vi "Keysight_ATI40_5.vi"() -> ()   [LabVIEW 2023]
uses:
  <vilib>/Analysis/baseanly.llb/A x Vector.vi
  <vilib>/Utility/file.llb/Write To Spreadsheet File (DBL).vi
  <instrlib>/Agilent 34970/Agilent 34970.lvlib
  <vilib>/Analysis/NI_AALBase.lvlib
panel:
  in  "Transform":T1
  in  "Torque Units":string="N-m"
  in  "Force Units":string="N"
  in  "Calibration File":path=path "C:/Users/d066566/OneDrive - Politecnico di Torino/PhD/PhD/Test files/Denver/FT17838/FT17838.cal"
  out "Output Number Array":dbl[](array[numeric]) format="%.2f"
  out "error out":errorcluster
  in  "Save":bool
  in  "Data File":path=path "C:/Users/d066566/Desktop/asdf3.csv"
  in  "Data format and type":string="%.6f"
  in  "stop":bool
  in  "VISA resource name":refnum<visa-resource-name>="GPIB0::9::INSTR"
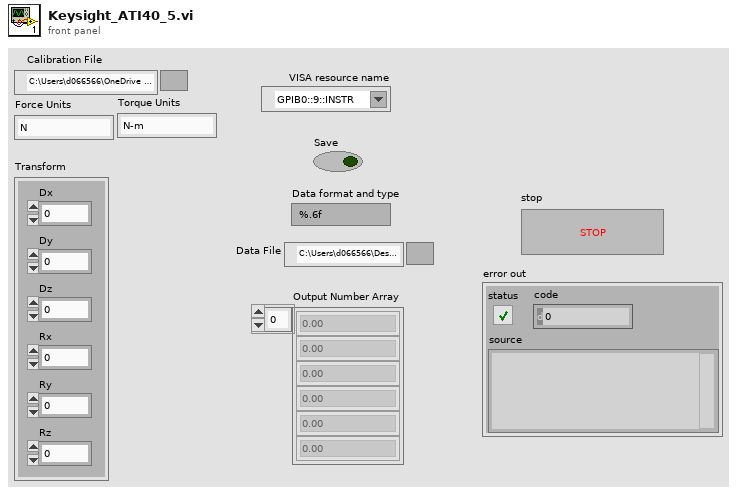
[diagram p1: front panel]
types:
  T1 = cluster{"Dx":dbl, "Dy":dbl, "Dz":dbl, "Rx":dbl, "Ry":dbl, "Rz":dbl}
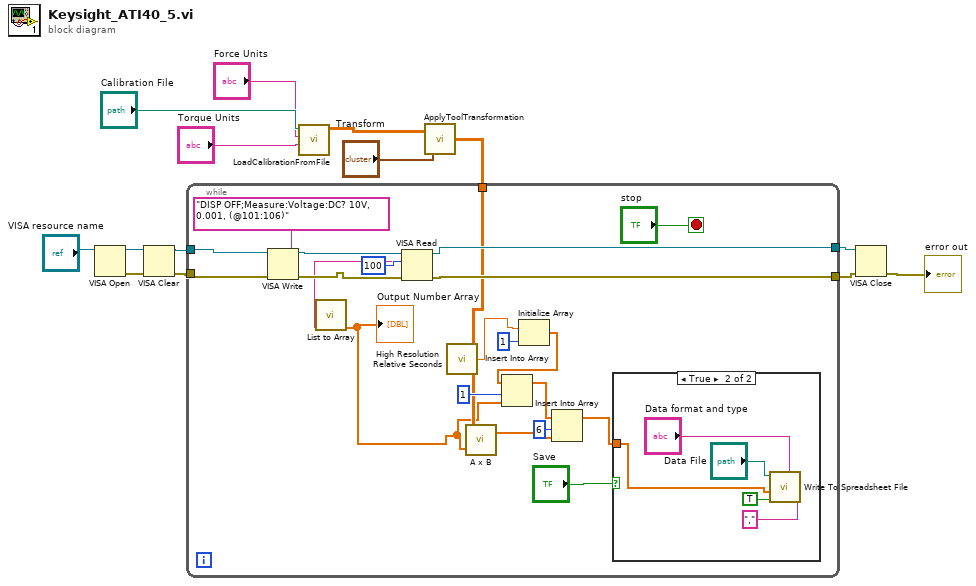
[diagram p0: block diagram]
diagram:
  n1 = VISA Open(VISA resource name="VISA resource name") -> (VISA resource name=w13:refnum<visa-resource-name>, error out=w12:errorcluster)  [unwired: 4 in]
  n2 = VISA Clear(VISA resource name=w13, error in (no error)=w12) -> (VISA resource name out=w8:refnum<visa-resource-name>, error out=w7:errorcluster)
  n3 = call "LoadCalibrationFromFile.vi"("User Torque Units"="Torque Units", "User Force Units"="Force Units", "Cal File Path"="Calibration File") -> ("Calibration Matrix"=w3:dbl[][])  [unwired: 1 in, 3 out]
  n4 = call "ApplyToolTransformation.vi"("Transform"="Transform", "Calibration Matrix"=w3) -> ("Transformed Calibration Matrix"=w1:dbl[][])
  n5 = while {
    tunnel: [w33] -> w11
    tunnel: [w32] -> w10
    tunnel: w7 -> [w25]
    tunnel: w8 -> [w24]
    tunnel: w1 -> [w23]
    stop <- "stop" stop-if-true
    n6 = VISA Write(VISA resource name=w24, write buffer="DISP OFF;Measure:Voltage:DC? 10V, 0.001, (@101:106)", error in (no error)=w25) -> (VISA resource name out=w29:refnum<visa-resource-name>, error out=w30:errorcluster)  [unwired: 1 out]
    n7 = VISA Read(VISA resource name=w29, byte count=u32 100, error in (no error)=w30) -> (VISA resource name out=w32:refnum<visa-resource-name>, read buffer=w28:string, error out=w33:errorcluster)  [unwired: 1 out]
    n8 = call <instrlib>:"List to Array.vi"("List (empty)"=w28) -> ("Output Number Array"=w17:dbl[])  [unwired: 9 in, 1 out]
    "Output Number Array" <- w17
    n9 = call <vilib>:"High Resolution Relative Seconds.vi"() -> ("relative seconds"=w19:dbl)
    n10 = call-poly <vilib>:"A x B.vi"("Vector"=w17, "A"=w23) -> ("A x Vector"=w21:dbl[])  [unwired: 1 out]
    n11 = Initialize Array(w19, 1 ("dimension size")) -> (w18:dbl[])
    n12 = Insert Into Array(array=w18, index=1, new element=w17) -> (w16:dbl[])
    n13 = Insert Into Array(array=w16, index=6, new element=w21) -> (w20:dbl[])
    n14 = case shown="True" "Save" {
      tunnel: w20 -> [_ w36]
      frame False {
      }
      frame True {
        n15 = call-poly <vilib>:"Write To Spreadsheet File.vi"("delimiter (\\t)"=",", "format (%.3f)"="Data format and type", "append to file? (new file:F)"=TRUE, "1D data"=w36, "file path (dialog if empty)"="Data File") -> ()  [unwired: 3 in, 1 out]
      }
    }
  }
  n16 = VISA Close(VISA resource name=w10, error in (no error)=w11) -> (error out=→"error out":errorcluster)
